vi "gaussian_fit.vi"(7 "expected size in pixels":dbl, 8 "error in (no error)":errorcluster, 10 "all rows":u16[][](array[numeric])) -> (0 "error out":errorcluster, 1 "best fit parameters":dbl[](array[numeric]), 2 "best fit image":dbl[][](graph))   [LabVIEW 2010]
uses:
  <vilib>/gmath/NumericalOptimization/LM model function reference.ctl
  <vilib>/gmath/NumericalOptimization/Nonlinear Curve Fit LM.vi
  <vilib>/gmath/NI_Gmath.lvlib
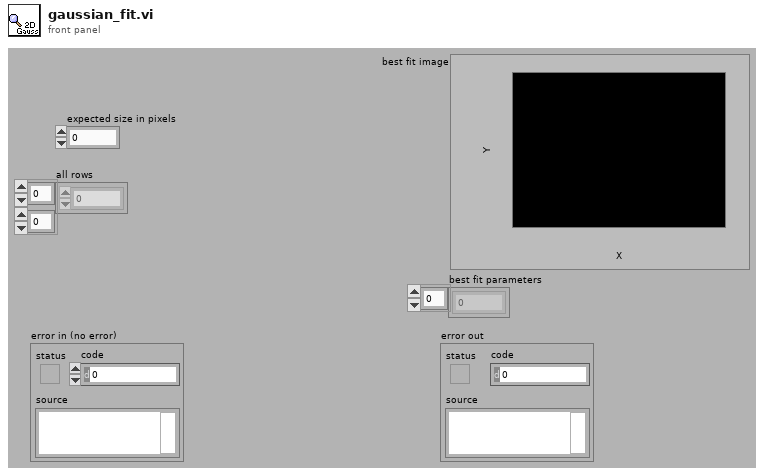
[diagram p1: front panel]
types:
  T1 = typedef "NI_Gmath.lvlib/LM model function reference.ctl" = refnum<vi>
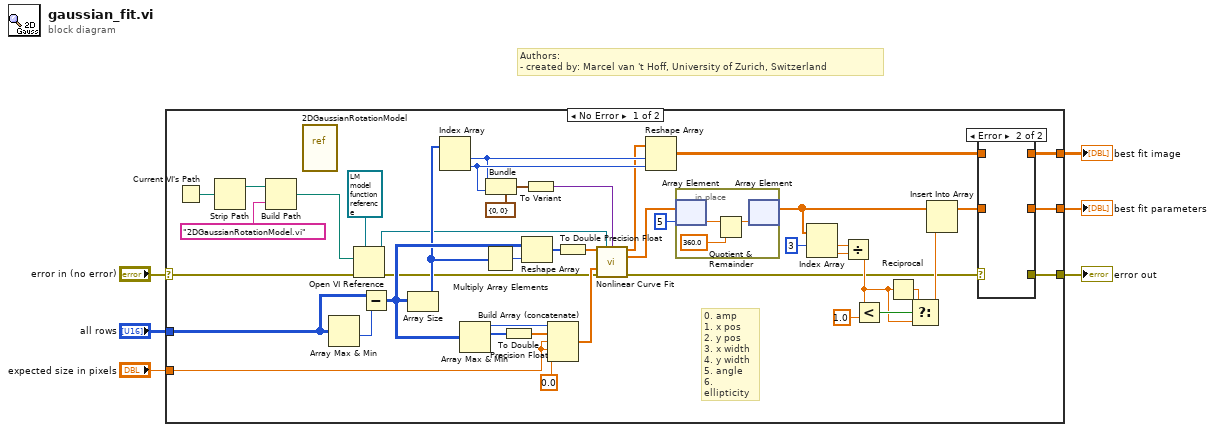
[diagram p0: block diagram]
diagram:
  # "Authors: \n- created by: Marcel van 't Hoff, University of Zurich, Switzerland"
  n1 = case shown="No Error" "error in (no error)" {
    selector: "error in (no error)" -> [w14 w57]
    tunnel: [w20 w57] -> w6
    tunnel: [w19 _] -> w1
    tunnel: [w17 _] -> w5
    tunnel: "expected size in pixels" -> [w39 _]
    tunnel: "all rows" -> [w33 _]
    frame No Error {
      # "0. amp\n1. x pos\n2. y pos\n3. x width\n4. y width\n5. angle\n6. ellipticity"
      n2 = Current VI's Path() -> (path=w11:path)
      n3 = Strip Path(path=w11) -> (stripped path=w10:path)  [unwired: 1 out]
      n4 = Build Path(base path=w10, name or relative path="2DGaussianRotationModel.vi") -> (appended path=w8:path)
      n5 = vi-ref "2DGaussianRotationModel.vi"() -> ()  [unwired: 1 out]
      n6 = Array Max & Min(array=w33) -> (min value=w50:u16)  [unwired: 3 out]
      n7 = Open VI Reference(type specifier VI Refnum (for type only)=T1 refnum ("f(x,a)"), vi path=w8, error in (no error)=w14) -> (vi reference=w15:T1, error out=w13:errorcluster)  [unwired: 3 in]
      n8 = Subtract(x=w33, y=w50) -> (x-y=w49:u16[][])
      n9 = Array Size(array=w49) -> (size(s)=w42:i32[])
      n10 = Index Array(array=w42) -> (element #1=w47:i32, element #2=w48:i32)  [unwired: 2 in]
      n11 = Array Max & Min(array=w49) -> (max value=w35:u16, max index (indices)=w36:i32[])  [unwired: 2 out]
      n12 = Multiply Array Elements(1:w42) -> (0:w34:i32)
      n13 = Bundle(cluster=cluster{"Width":i32, "Height":i32} {"Width"=0, "Height"=0} ("Plot Area:Size"), "Width"=w47, "Height"=w48) -> (w45:cluster{"Width":i32, "Height":i32})
      n14 = To Double Precision Float(number=w36) -> (double precision float=w37:dbl[])
      n15 = Reshape Array(w49, w34) -> (w38:u16[])
      n16 = To Variant(anything=w45) -> (Variant=w46:variant)
      n17 = Build Array (concatenate)(w35, w37, w39, w39, 0.0 ("element")) -> (w41:dbl[])
      n18 = To Double Precision Float(number=w38) -> (double precision float=w7:dbl[])
      n19 = call-poly <vilib>:"Nonlinear Curve Fit.vi"("Y"=w7, "f(x,a)"=w15, "data"=w46, "initial parameters"=w41, "error in (no error)"=w13) -> ("best nonlinear fit"=w43:dbl[], "best fit parameters"=w32:dbl[], "error out"=w21:errorcluster)  [unwired: 5 in, 3 out]
      n20 = Reshape Array(w43, w47, w48) -> (w18:dbl[][])
      n21 = in-place {
        n22 = in-place-array #1(w32, 5) -> (w56:dbl)
        n23 = Quotient & Remainder(x=w56, y=360.0) -> (x-y*floor(x/y)=w54:dbl)  [unwired: 1 out]
        n24 = in-place-array #1(w54) -> (w30:dbl[])  [unwired: 1 out]
      }
      n25 = Index Array(array=w30, index #1=3 ("index")) -> (element #1=w28:dbl, element #2=w27:dbl)  [unwired: 1 in]
      n26 = Divide(x=w28, y=w27) -> (x/y=w23:dbl)
      n27 = Less?(x=w23, y=1.0 ("x")) -> (x < y?=w26:bool)
      n28 = Reciprocal(x=w23) -> (1/x=w24:dbl)
      n29 = Select(t=w24, s=w26, f=w23) -> (s? t:f=w22:dbl)
      n30 = Insert Into Array(array=w30, new element=w22) -> (w16:dbl[])  [unwired: 1 in]
      n31 = case shown="Error" w21 {
        selector: w21 -> [w53 _]
        tunnel: [w53 _] -> w20
        tunnel: [w52 _] -> w19
        tunnel: w18 -> [w52 _]
        tunnel: [w51 _] -> w17
        tunnel: w16 -> [w51 _]
        frame No Error {
        }
        frame Error {
        }
      }
    }
    frame Error {
    }
  }
  "error out" <- w6
  "best fit parameters" <- w5
  "best fit image" <- w1
